vi "Compare Character Types.vi"() -> ()   [LabVIEW 2023]
doc: "This examples demonstrates the functionality of the character comparison functions. These functions include Decimal Digit?, Hex Digit?, Octal Digit?, Printable?, White Space?, and Lexical Class."
panel:
  in  "Stop":bool
  out "class number":i16
  out "space, h/v tab, cr, lf, ff?":bool
  out "printable ASCII?":bool
  out "octal?":bool
  out "hex?":bool
  out "digit?":bool
  in  "Character":string="A"
  # "Overview: Demonstrates the functionality of the character comparison functions. These functions include Decimal Digit?, Hex Digit?, Octal Digit?, Printable?, White Space?, and Lexical Class.\nInstructions:\n1. Run the VI.\n2. Enter a single character in the Character string and observe the results of the character comparison.\n3. Try several different characters and observe the results.\n4. Click Stop to stop the VI."
  # "The character comparison functions only look at the first character in the char string."
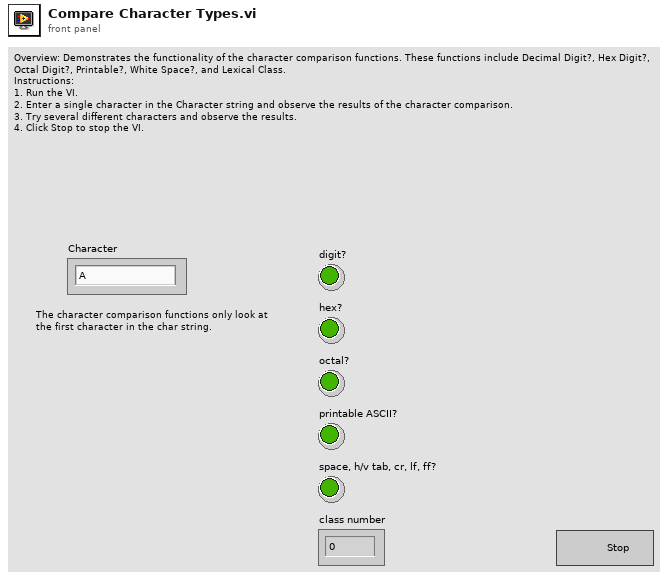
[diagram p1: front panel]
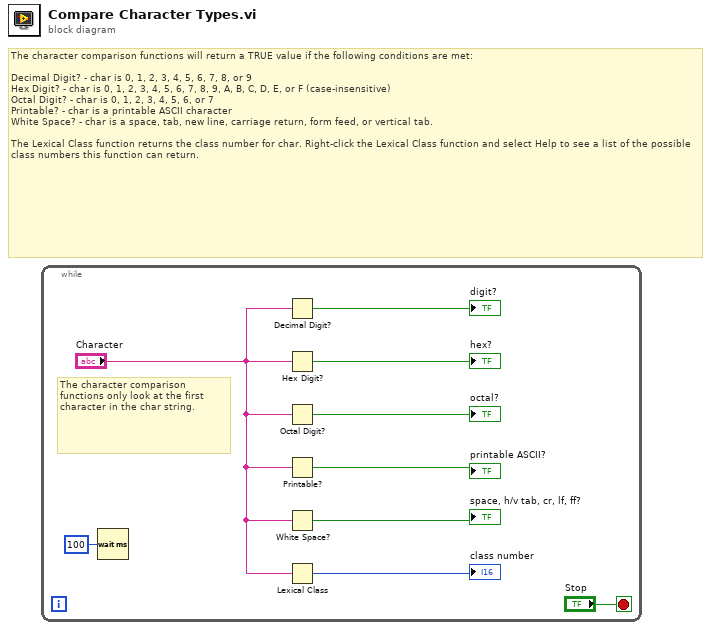
[diagram p0: block diagram]
diagram:
  # "The character comparison functions will return a TRUE value if the following conditions are met:\n\nDecimal Digit? - char is 0, 1, 2, 3, 4, 5, 6, 7, 8, or 9\nHex Digit? - char is 0, 1, 2, 3, 4, 5, 6, 7, 8, 9, A, B, C, D, E, or F (case-insensitive)\nOctal Digit? - char is 0, 1, 2, 3, 4, 5, 6, or 7\nPrintable? - char is a printable ASCII character\nWhite Space? - char is a space, tab, new line, carriage return, form feed, or vertical tab.\n\nThe Lexical Class function returns the class number for char. Right-click the Lexical Class function and select Help to see a list of the possible class numbers this function can return."
  n1 = while {
    stop <- "Stop" stop-if-true
    # "The character comparison functions only look at the first character in the char string."
    n2 = Wait (ms)(milliseconds to wait=u32 100) -> ()  [unwired: 1 out]
    n3 = Decimal Digit?(1:"Character") -> (0:→"digit?":bool)
    n4 = Hex Digit?(1:"Character") -> (0:→"hex?":bool)
    n5 = Octal Digit?(1:"Character") -> (0:→"octal?":bool)
    n6 = Printable?(1:"Character") -> (0:→"printable ASCII?":bool)
    n7 = White Space?(1:"Character") -> (0:→"space, h/v tab, cr, lf, ff?":bool)
    n8 = Lexical Class(1:"Character") -> (0:→"class number":i16)
  }
